vi "File_Check Valid.vi"(0 "path":path) -> (2 "No Path":bool, 4 "dup path":path, 5 "valid":bool)   [LabVIEW 2020]
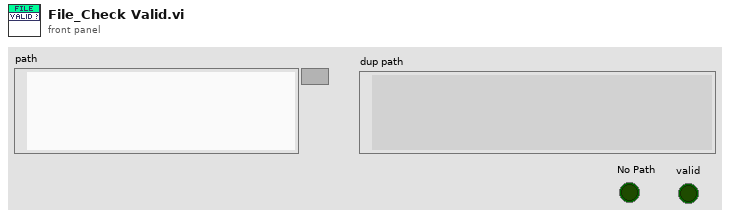
[diagram p1: front panel]
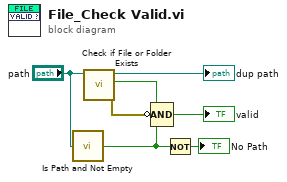
[diagram p0: block diagram]
diagram:
  n1 = call <vilib>:"Is Path and Not Empty.vi"("path"="path") -> ("Is Path and Not Empty?"=w2:bool)  [unwired: 4 in]
  n2 = call <vilib>:"Check if File or Folder Exists.vi"("path"="path") -> ("error out"=w4:errorcluster, "file or folder exists?"=w5:bool, "dup path"=→"dup path":path)  [unwired: 8 in]
  n3 = Compound Arithmetic op=AND(w5, invert w4, w2) -> (→"valid":bool)
  n4 = Not(x=w2) -> (.not. x?=→"No Path":bool)
